vi "SafeOpenPins (SubVI).vi"(0 "LakeshoreVISA Refnum in":refnum<visa-resource-name>, 1 "Settings array in":i32[](array[numeric]), 5 "error in (no error)":errorcluster, 7 "Channel Str":string, 9 "Switchboard VISA Refnum in":refnum<visa-resource-name>, 11 "Switchboard error in":errorcluster) -> (3 "Settings array out":i32[](array[numeric]), 4 "VISA Refnum out":refnum<visa-resource-name>, 6 "error out":errorcluster, 10 "VISA resource name out":refnum<visa-resource-name>, 15 "Switchboard error out":errorcluster)   [LabVIEW 2017, in "Fridge Software v2.1.lvlib"]
uses:
  Fridge Software v2.1.lvlib
  <instrlib>/Keithley 3706/Keithley 3700 Series.lvlib
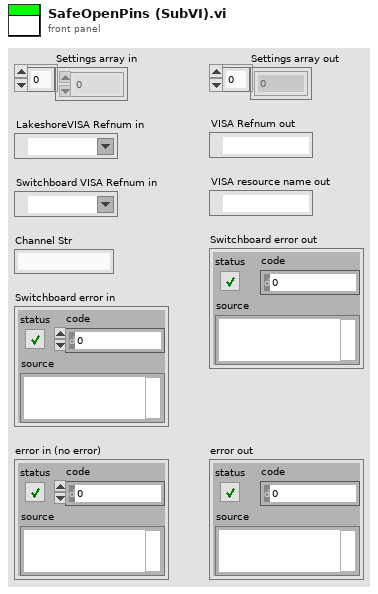
[diagram p1: front panel]
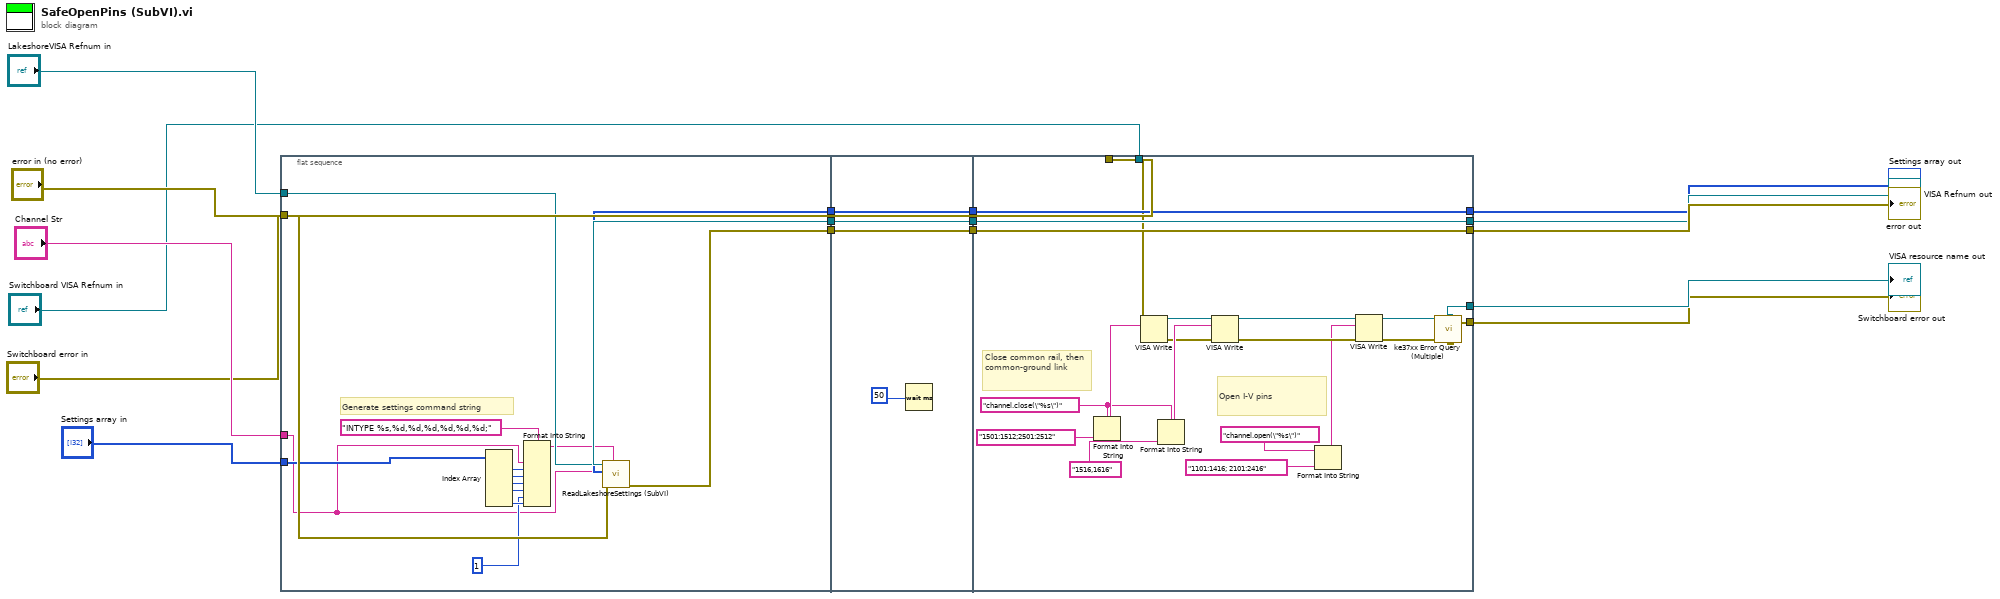
[diagram p0: block diagram]
diagram:
  n1 = flat-sequence {
    tunnel: "error in (no error)" -> [w31]
    tunnel: "LakeshoreVISA Refnum in" -> [w29]
    tunnel: "Settings array in" -> [w27]
    tunnel: "Channel Str" -> [w18]
    tunnel: [w32] -> w6
    tunnel: [w30] -> w4
    tunnel: [w28] -> w2
    tunnel: w6 -> [w36]
    tunnel: [w36] -> w5
    tunnel: w4 -> [w35]
    tunnel: [w35] -> w3
    tunnel: w2 -> [w34]
    tunnel: [w34] -> w1
    tunnel: [w55] -> w11
    tunnel: [w37] -> w12
    tunnel: [w38] -> w13
    tunnel: [w56] -> w15
    tunnel: [w57] -> w17
    tunnel: w5 -> [w57]
    tunnel: w3 -> [w56]
    tunnel: w1 -> [w55]
    tunnel: "Switchboard error in" -> [w40]
    tunnel: "Switchboard VISA Refnum in" -> [w39]
    frame #0 {
      # "Generate settings command string"
      n2 = Index Array(array=w27) -> (element #1=w21:i32, element #2=w22:i32, element #3=w23:i32, element #4=w24:i32, element #6=w25:i32)  [unwired: 6 in, 1 out]
      n3 = Format Into String(format string="INTYPE %s,%d,%d,%d,%d,%d,%d;", w18, w21, w22, w23, w24, 1, w25) -> (resulting string=w26:string)  [unwired: 2 in, 1 out]
      n4 = call "ReadLakeshoreSettings (SubVI).vi"("Prepended command"=w26, "error in (no error)"=w31, "Channel Str"=w18, "Lakeshore port"=w29) -> ("error out"=w32:errorcluster, "Settings array out"=w28:i32[], "VISA Refnum out"=w30:refnum<visa-resource-name>)  [unwired: 3 in]
    }
    frame #1 {
      n5 = Wait (ms)(milliseconds to wait=50) -> ()  [unwired: 1 out]
    }
    frame #2 {
      w43 = "channel.close(\"%s\")"
      # "Open I-V pins"
      # "Close common rail, then common-ground link"
      n6 = Format Into String(format string=w43, "1501:1512;2501:2512") -> (resulting string=w54:string)  [unwired: 2 in, 1 out]
      n7 = VISA Write(VISA resource name=w39, write buffer=w54, error in (no error)=w40) -> (VISA resource name out=w52:refnum<visa-resource-name>, error out=w51:errorcluster)  [unwired: 1 out]
      n8 = Format Into String(format string=w43, "1516,1616") -> (resulting string=w53:string)  [unwired: 2 in, 1 out]
      n9 = VISA Write(VISA resource name=w52, write buffer=w53, error in (no error)=w51) -> (VISA resource name out=w50:refnum<visa-resource-name>, error out=w49:errorcluster)  [unwired: 1 out]
      n10 = Format Into String(format string="channel.open(\"%s\")", "1101:1416; 2101:2416") -> (resulting string=w48:string)  [unwired: 2 in, 1 out]
      n11 = VISA Write(VISA resource name=w50, write buffer=w48, error in (no error)=w49) -> (VISA resource name out=w47:refnum<visa-resource-name>, error out=w46:errorcluster)  [unwired: 1 out]
      n12 = call <instrlib>:"ke37xx Error Query (Multiple).vi"("VISA resource name"=w47, "error in (no error)"=w46) -> ("VISA resource name out"=w38:refnum<visa-resource-name>, "error out"=w37:errorcluster)  [unwired: 10 in, 2 out]
    }
  }
  "error out" <- w17
  "VISA Refnum out" <- w15
  "VISA resource name out" <- w13
  "Switchboard error out" <- w12
  "Settings array out" <- w11
